vi "Shutdown All Processes.vi"(8 "Error In":errorcluster, 11 "Error Handling In":refnum<class "Error Handling.lvclass">) -> (0 "Error Out":errorcluster, 3 "Error Handling Out":refnum<class "Error Handling.lvclass">)   [LabVIEW 2021, in "Error Handling.lvclass"]
uses:
  Error Handling.lvclass
  C:/Git/MEMOSFET/myDashBoard/Source/RT/Process/Process.lvclass
  Central Message Handler/Public/Controls/Message.ctl
  Process/Accessors/Central Message Handler Queue/Get Central Message Handler Queue.vi
  Central Message Handler/Central Message Handler.lvclass
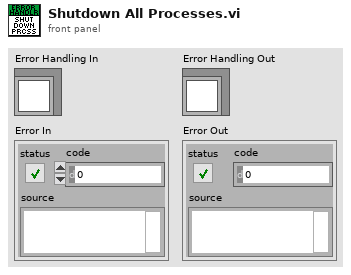
[diagram p1: front panel]
types:
  T1 = typedef "Central Message Handler.lvclass/Message.ctl" = cluster{"Command":string, "Data":variant, "Receiver":string}
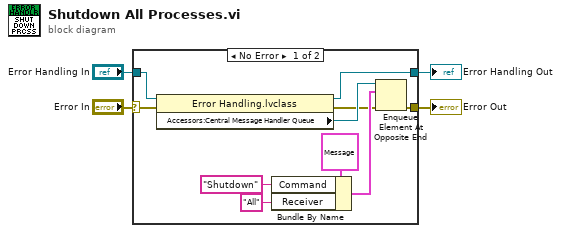
[diagram p0: block diagram]
diagram:
  n1 = case shown="No Error" "Error In" {
    selector: "Error In" -> [w11 w15]
    tunnel: [w14 w15] -> w4
    tunnel: [w13 w16] -> w3
    tunnel: "Error Handling In" -> [w12 w16]
    frame No Error {
      n2 = property class="Error Handling.lvclass"(reference=w12, error in=w11) -> (reference out=w13:refnum<class "Error Handling.lvclass">, error out=w5:errorcluster, "Accessors:Central Message Handler Queue"=w6:refnum<queue>)
      n3 = Bundle By Name(cluster=T1 {"Command"="", "Data"=variant, "Receiver"=""} ("element"), "Command"="Shutdown", "Receiver"="All") -> (w10:T1)
      n4 = Enqueue Element At Opposite End(queue=w6, element=w10, error in (no error)=w5) -> (error out=w14:errorcluster)  [unwired: 1 in, 2 out]
    }
    frame Error {
    }
  }
  "Error Out" <- w4
  "Error Handling Out" <- w3
